vi "Write Controls to Config File.vi"(6 "Child?":bool, 7 "section":string, 8 "Error In":errorcluster, 9 "ParentName":string, 10 "Ctl Refnum":refnum<vi>, 11 "refnum":T1) -> (0 "Error Out":errorcluster, 3 "refnum out":T1)   [LabVIEW 2018]
uses:
  <vilib>/Utility/config.llb/Config Data RefNum.ctl
  Hardware Mfg/Thorlabs Translation Stages/Controls/Translation Stage Cluster.ctl
  Controls/Translation Stage Types.ctl
  <vilib>/Utility/config.llb/Write Key (String).vi
  <vilib>/Utility/config.llb/Write Key (Path).vi
  <vilib>/Utility/config.llb/Write Key (Boolean).vi
  <vilib>/Utility/config.llb/Write Key (Double).vi
  <vilib>/Utility/config.llb/Write Key (U32).vi
  <vilib>/Utility/config.llb/NI_LVConfig.lvlib
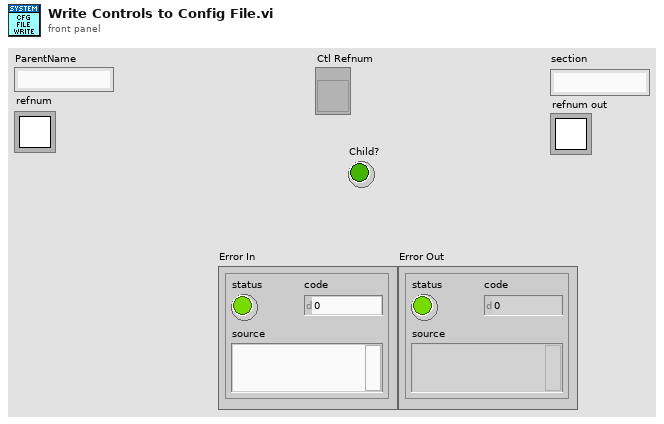
[diagram p1: front panel]
types:
  T1 = typedef "NI_LVConfig.lvlib/Config Data RefNum.ctl" = refnum<k1>
  T2 = typedef "Translation Stage Cluster.ctl" = cluster{"Position":dbl, "Is.Enabled?":bool, "Is.Connected?":bool, "Device SN":string, "AccelerationMaximum":dbl, "VelocityMaximum":dbl, "Acceleration":dbl, "Velocity":dbl, "waitTimeout (ms)":i32, "Model":T3, "Is.Homed?":bool}
  T3 = typedef "Translation Stage Types.ctl" = enum16{"None", "Thorlabs LTS", "Thorlabs MLJ"}
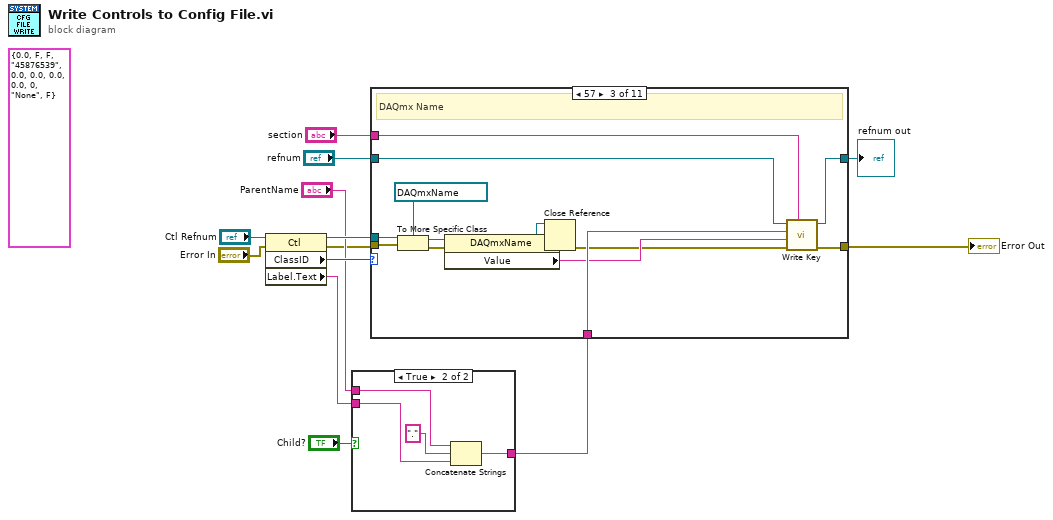
[diagram p0: block diagram]
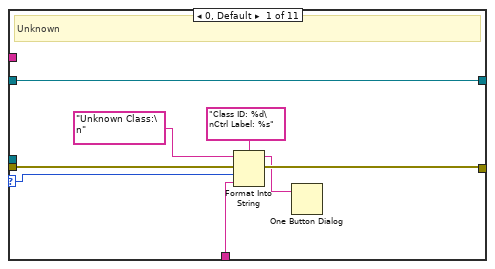
[diagram p3: hidden frame]
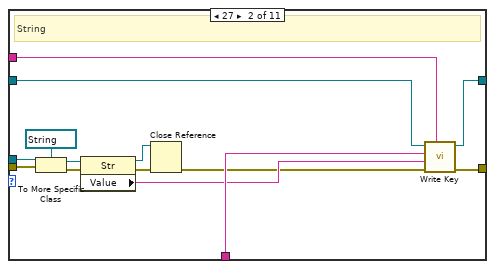
[diagram p4: hidden frame]
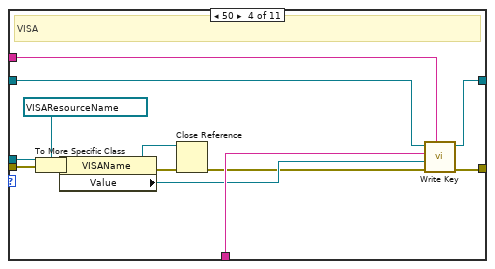
[diagram p5: hidden frame]
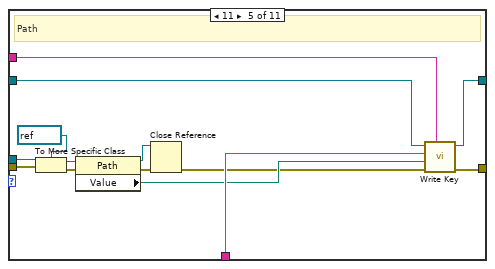
[diagram p6: hidden frame]
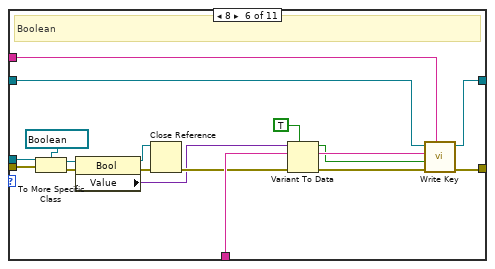
[diagram p7: hidden frame]
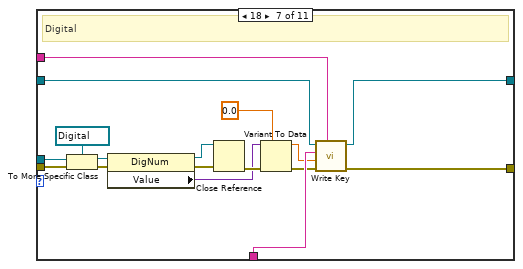
[diagram p8: hidden frame]
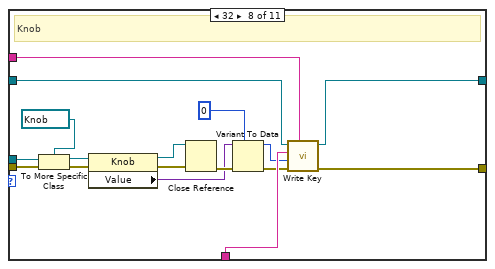
[diagram p9: hidden frame]
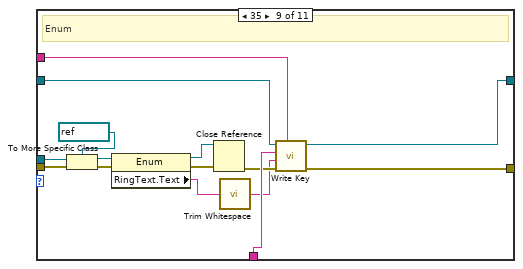
[diagram p10: hidden frame]
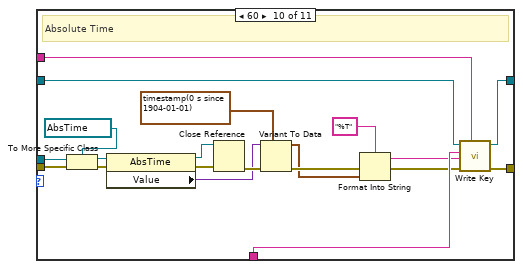
[diagram p11: hidden frame]
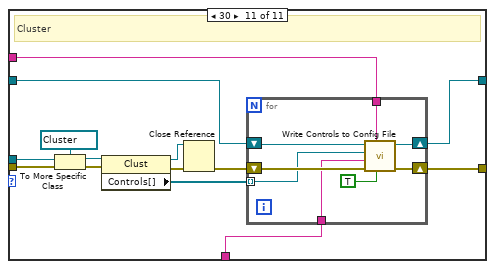
[diagram p12: hidden frame]
diagram:
  (unwired) T2 {"Position"=0.0, "Is.Enabled?"=FALSE, "Is.Connected?"=FALSE, "Device SN"="45876539", "AccelerationMaximum"=0.0, "VelocityMaximum"=0.0, "Acceleration"=0.0, "Velocity"=0.0, "waitTimeout (ms)"=0, "Model"=enum."None", "Is.Homed?"=FALSE} ("Control Param In")
  n1 = property class="Ctl"(reference="Ctl Refnum", error in="Error In") -> (reference out=w12:refnum<vi>, error out=w6:errorcluster, "ClassID"=w11:u32, "Label.Text"=w8:string)
  n2 = case shown="True" "Child?" {
    tunnel: "ParentName" -> [_ w18]
    tunnel: w8 -> [w14 w16]
    tunnel: [w14 w15] -> w3
    frame False {
    }
    frame True {
      n3 = Concatenate Strings(w18, ".", w16) -> (w15:string)
    }
  }
  n4 = case shown="57" w11 {
    selector: w11 -> [w23 _ _ _ _ _ _ _ _ _ _]
    tunnel: w6 -> [w21 w39 w54 w68 w82 w98 w116 w133 w148 w168 w182]
    tunnel: w12 -> [_ w38 w53 w67 w81 w97 w115 w132 w147 w167 w180]
    tunnel: [w20 w37 w52 w66 w80 w96 w104 w122 w138 w157 w176] -> w1
    tunnel: "section" -> [_ w36 w51 w65 w79 w95 w107 w125 w141 w160 w173]
    tunnel: "refnum" -> [w26 w35 w50 w64 w78 w94 w106 w124 w140 w159 w175]
    tunnel: [w26 w34 w49 w63 w77 w93 w105 w123 w139 w158 w174] -> w2
    tunnel: w3 -> [w22 w32 w47 w61 w75 w91 w108 w126 w142 w161 w172]
    frame 0, Default {
      # "Unknown"
      n5 = Format Into String(format string="Class ID: %d\nCtrl Label: %s", initial string="Unknown Class:\n" ("string"), error in=w21, w23, w22) -> (resulting string=w19:string, error out=w20:errorcluster)
      n6 = One Button Dialog(message=w19) -> ()  [unwired: 1 in, 1 out]
    }
    frame 27 {
      # "String"
      n7 = To More Specific Class(target class=refnum<vi> refnum ("AccelerationMaximum 2"), reference=w38, error in=w39) -> (specific class reference=w30:refnum<vi>, error out=w33:errorcluster)
      n8 = property class="Str"(reference=w30, error in=w33) -> (reference out=w27:refnum<vi>, error out=w31:errorcluster, "Value"=w29:string)
      n9 = Close Reference(reference=w27, error in (no error)=w31) -> (error out=w28:errorcluster)
      n10 = call-poly <vilib>:"Write Key.vi"("section"=w36, "error in (no error)"=w28, "value"=w29, "key"=w32, "refnum"=w35) -> ("error out"=w37:errorcluster, "refnum out"=w34:T1)  [unwired: 4 in, 1 out]
    }
    frame 57 {
      # "DAQmx Name"
      n11 = To More Specific Class(target class=refnum<vi> refnum ("Analog Out Channel"), reference=w53, error in=w54) -> (specific class reference=w45:refnum<vi>, error out=w48:errorcluster)
      n12 = property class="DAQmxName"(reference=w45, error in=w48) -> (reference out=w42:refnum<vi>, error out=w46:errorcluster, "Value"=w44:string)
      n13 = Close Reference(reference=w42, error in (no error)=w46) -> (error out=w43:errorcluster)
      n14 = call-poly <vilib>:"Write Key.vi"("section"=w51, "error in (no error)"=w43, "value"=w44, "key"=w47, "refnum"=w50) -> ("error out"=w52:errorcluster, "refnum out"=w49:T1)  [unwired: 4 in, 1 out]
    }
    frame 50 {
      # "VISA"
      n15 = To More Specific Class(target class=refnum<vi> refnum ("Controller VISA Ref"), reference=w67, error in=w68) -> (specific class reference=w59:refnum<vi>, error out=w62:errorcluster)
      n16 = property class="VISAName"(reference=w59, error in=w62) -> (reference out=w56:refnum<vi>, error out=w60:errorcluster, "Value"=w58:refnum<visa-resource-name>)
      n17 = Close Reference(reference=w56, error in (no error)=w60) -> (error out=w57:errorcluster)
      n18 = call-poly <vilib>:"Write Key.vi"("section"=w65, "error in (no error)"=w57, "value"=w58, "key"=w61, "refnum"=w64) -> ("error out"=w66:errorcluster, "refnum out"=w63:T1)  [unwired: 4 in, 1 out]
    }
    frame 11 {
      # "Path"
      n19 = To More Specific Class(target class=refnum<vi> refnum ("Path"), reference=w81, error in=w82) -> (specific class reference=w73:refnum<vi>, error out=w76:errorcluster)
      n20 = property class="Path"(reference=w73, error in=w76) -> (reference out=w70:refnum<vi>, error out=w74:errorcluster, "Value"=w72:path)
      n21 = Close Reference(reference=w70, error in (no error)=w74) -> (error out=w71:errorcluster)
      n22 = call-poly <vilib>:"Write Key.vi"("section"=w79, "error in (no error)"=w71, "value"=w72, "key"=w75, "refnum"=w78) -> ("error out"=w80:errorcluster, "refnum out"=w77:T1)  [unwired: 4 in, 1 out]
    }
    frame 8 {
      # "Boolean"
      n23 = To More Specific Class(target class=refnum<vi> refnum ("AccelerationMaximum 2"), reference=w97, error in=w98) -> (specific class reference=w89:refnum<vi>, error out=w92:errorcluster)
      n24 = property class="Bool"(reference=w89, error in=w92) -> (reference out=w87:refnum<vi>, error out=w90:errorcluster, "Value"=w85:variant)
      n25 = Close Reference(reference=w87, error in (no error)=w90) -> (error out=w88:errorcluster)
      n26 = Variant To Data(error in=w88, type=TRUE, Variant=w85) -> (data=w83:bool, error out=w86:errorcluster)
      n27 = call-poly <vilib>:"Write Key.vi"("section"=w95, "error in (no error)"=w86, "value"=w83, "key"=w91, "refnum"=w94) -> ("error out"=w96:errorcluster, "refnum out"=w93:T1)  [unwired: 4 in, 1 out]
    }
    frame 18 {
      # "Digital"
      n28 = To More Specific Class(target class=refnum<vi> refnum ("AccelerationMaximum 2"), reference=w115, error in=w116) -> (specific class reference=w112:refnum<vi>, error out=w113:errorcluster)
      n29 = property class="DigNum"(reference=w112, error in=w113) -> (reference out=w110:refnum<vi>, error out=w111:errorcluster, "Value"=w102:variant)
      n30 = Close Reference(reference=w110, error in (no error)=w111) -> (error out=w109:errorcluster)
      n31 = Variant To Data(error in=w109, type=0.0, Variant=w102) -> (data=w100:dbl, error out=w103:errorcluster)
      n32 = call-poly <vilib>:"Write Key.vi"("section"=w107, "error in (no error)"=w103, "value"=w100, "key"=w108, "refnum"=w106) -> ("error out"=w104:errorcluster, "refnum out"=w105:T1)  [unwired: 4 in, 1 out]
    }
    frame 32 {
      # "Knob"
      n33 = To More Specific Class(target class=refnum<vi> refnum ("Zoom Factor"), reference=w132, error in=w133) -> (specific class reference=w130:refnum<vi>, error out=w131:errorcluster)
      n34 = property class="Knob"(reference=w130, error in=w131) -> (reference out=w128:refnum<vi>, error out=w129:errorcluster, "Value"=w120:variant)
      n35 = Close Reference(reference=w128, error in (no error)=w129) -> (error out=w127:errorcluster)
      n36 = Variant To Data(error in=w127, type=u32 0, Variant=w120) -> (data=w118:u32, error out=w121:errorcluster)
      n37 = call-poly <vilib>:"Write Key.vi"("section"=w125, "error in (no error)"=w121, "value"=w118, "key"=w126, "refnum"=w124) -> ("error out"=w122:errorcluster, "refnum out"=w123:T1)  [unwired: 4 in, 1 out]
    }
    frame 35 {
      # "Enum"
      n38 = To More Specific Class(target class=refnum<vi> refnum ("Enum"), reference=w147, error in=w148) -> (specific class reference=w145:refnum<vi>, error out=w146:errorcluster)
      n39 = property class="Enum"(reference=w145, error in=w146) -> (reference out=w143:refnum<vi>, error out=w144:errorcluster, "RingText.Text"=w135:string)
      n40 = Close Reference(reference=w143, error in (no error)=w144) -> (error out=w136:errorcluster)
      n41 = call <vilib>:"Trim Whitespace.vi"("string"=w135) -> ("trimmed string"=w134:string)  [unwired: 1 in]
      n42 = call-poly <vilib>:"Write Key.vi"("section"=w141, "error in (no error)"=w136, "value"=w134, "key"=w142, "refnum"=w140) -> ("error out"=w138:errorcluster, "refnum out"=w139:T1)  [unwired: 4 in, 1 out]
    }
    frame 60 {
      # "Absolute Time"
      n43 = To More Specific Class(target class=refnum<vi> refnum ("AccelerationMaximum 2"), reference=w167, error in=w168) -> (specific class reference=w165:refnum<vi>, error out=w166:errorcluster)
      n44 = property class="AbsTime"(reference=w165, error in=w166) -> (reference out=w163:refnum<vi>, error out=w164:errorcluster, "Value"=w155:variant)
      n45 = Close Reference(reference=w163, error in (no error)=w164) -> (error out=w162:errorcluster)
      n46 = Variant To Data(error in=w162, type=timestamp(0 s since 1904-01-01), Variant=w155) -> (data=w149:timestamp, error out=w156:errorcluster)
      n47 = Format Into String(format string="%T", error in=w156, w149) -> (resulting string=w153:string, error out=w154:errorcluster)  [unwired: 1 in]
      n48 = call-poly <vilib>:"Write Key.vi"("section"=w160, "error in (no error)"=w154, "value"=w153, "key"=w161, "refnum"=w159) -> ("error out"=w157:errorcluster, "refnum out"=w158:T1)  [unwired: 4 in, 1 out]
    }
    frame 30 {
      # "Cluster"
      n49 = To More Specific Class(target class=refnum<vi> refnum ("Cluster Ref In"), reference=w180, error in=w182) -> (specific class reference=w178:refnum<vi>, error out=w179:errorcluster)
      n50 = property class="Clust"(reference=w178, error in=w179) -> (reference out=w170:refnum<vi>, error out=w177:errorcluster, "Controls[]"=w169:refnum<vi>[])
      n51 = Close Reference(reference=w170, error in (no error)=w177) -> (error out=w171:errorcluster)
      n52 = for {
        tunnel: w173 -> [w186]
        tunnel: w172 -> [w185]
        shift-right: [w189] -> w176
        shift-left: w171 -> [w190]
        shift-right: [w187] -> w174
        shift-left: w175 -> [w188]
        tunnel: w169 -> [w183] mode=indexing
        n53 = call "Write Controls to Config File.vi"("Child?"=TRUE, "section"=w186, "Error In"=w190, "ParentName"=w185, "Ctl Refnum"=w183, "refnum"=w188) -> ("Error Out"=w189:errorcluster, "refnum out"=w187:T1)  [unwired: 4 in]
      }
    }
  }
  "Error Out" <- w1
  "refnum out" <- w2
